vi "uPublisher BatchPublish.vi"(8 "error in (no error)":errorcluster, 10 "uMsgs":refnum<class "uMsg.lvclass">[](array[class]), 11 "uClient_Publisher in":refnum<class "uClient_Publisher.lvclass">) -> (0 "error out":errorcluster, 3 "uClient_Publisher out":refnum<class "uClient_Publisher.lvclass">)   [LabVIEW 2023, in "uLib.lvlib" / "uClient_Publisher.lvclass"]
doc: "Publish a batch of event to the broker in performance optimized manner."
uses:
  uClient_Publisher.lvclass
  uMsg/uMsg/uMsg.lvclass
  uClient_Publisher.lvclass/uClient_Publisher.ctl
  uData/uData/uData.lvclass
  uMsg/uMsg/uMsg.lvclass/uMsg.ctl
  uData/uData/uData.lvclass/uData.ctl
  uData/uData/Condition Tag Name.vi
  uData/uData/Blank Key Reserved String.vi
  uTransport/uTransport/uTransport.lvclass
  uStringManipulation/uStringManipulation/uStringManipulation.lvclass
  U:/Projects/uLib/Src/uFramework/uClient/uClient.lvclass
  U:/Projects/uLib/Src/uFramework/uClient_Publisher/uClient_Publisher.lvclass
  U:/Projects/uLib/Src/uFramework/uTransport/uTransport.lvclass
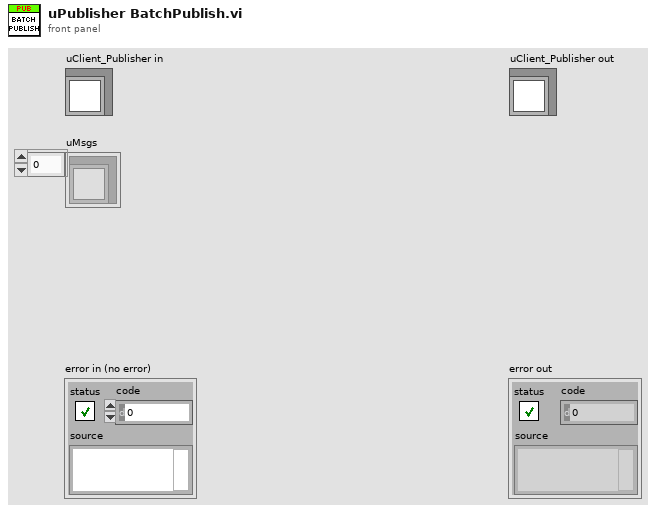
[diagram p1: front panel]
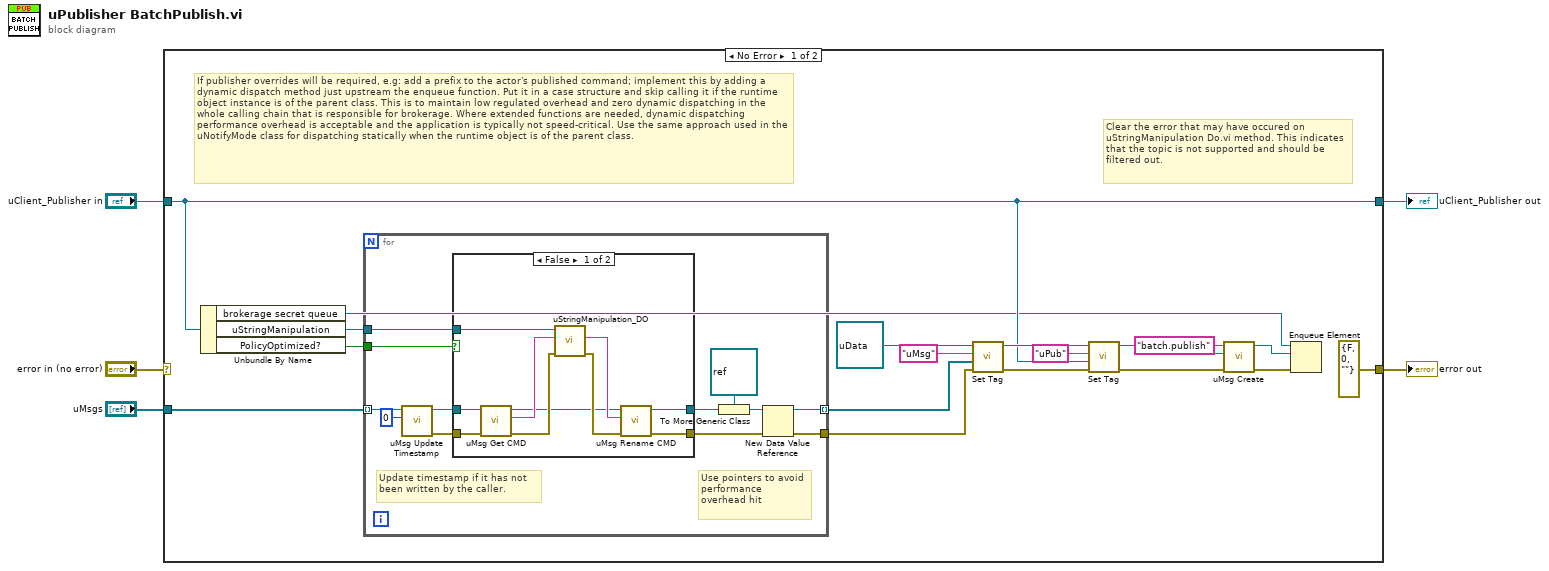
[diagram p0: block diagram]
diagram:
  n1 = case shown="No Error" "error in (no error)" {
    selector: "error in (no error)" -> [_ w48]
    tunnel: [errorcluster {"status"=FALSE, "code"=0, "source"=""} ("error IO") w48] -> w5
    tunnel: "uClient_Publisher in" -> [w12 w49]
    tunnel: "uMsgs" -> [w7 _]
    tunnel: [w12 w49] -> w2
    frame No Error {
      # "Clear the error that may have occured on uStringManipulation Do.vi method. This indicates that the topic is not supported and should be filtered out."
      # "If publisher overrides will be required, e.g: add a prefix to the actor's published command; implement this by adding a dynamic dispatch method just upstream the enqueue function. Put it in a case structure and skip calling it if the runtime object instance is of the parent class. This is to maintain low regulated overhead and zero dynamic dispatching in the whole calling chain that is responsible for brokerage. Where extended functions are needed, dynamic dispatching performance overhead is acceptable and the application is typically not speed-critical. Use the same approach used in the uNotifyMode class for dispatching statically when the runtime object is of the parent class."
      n2 = Unbundle By Name(w12) -> ("brokerage secret queue"=w6:refnum<queue>, "uStringManipulation"=w13:refnum<class "uStringManipulation.lvclass">, "PolicyOptimized?"=w8:bool)
      n3 = for {
        tunnel: [w35] -> w15
        tunnel: [w28] -> w14 mode=indexing
        tunnel: w13 -> [w34]
        tunnel: w8 -> [w33]
        tunnel: w7 -> [w30] mode=indexing
        # "Use pointers to avoid performance overhead hit"
        # "Update timestamp if it has not been written by the caller."
        n4 = call "uMsg Update Timestamp.vi"("Timestamp"=u32 0, "uMsg in"=w30) -> ("error out"=w29:errorcluster, "uMsg out"=w31:refnum<class "uMsg.lvclass">)  [unwired: 8 in]
        n5 = case shown="False" w33 {
          tunnel: w34 -> [w45 _]
          tunnel: w31 -> [w42 w47]
          tunnel: [w43 w47] -> w27
          tunnel: w29 -> [w38 w46]
          tunnel: [w36 w46] -> w24
          frame False {
            n6 = call "uMsg Get CMD.vi"("error in (no error)"=w38, "uMsg in"=w42) -> ("error out"=w41:errorcluster, "CMD"=w39:string, "uMsg out"=w37:refnum<class "uMsg.lvclass">)  [unwired: 7 in]
            n7 = call-dynamic "uStringManipulation_DO.vi"("error in (no error)"=w41, "String in"=w39, "uStringManipulation in"=w45) -> ("error out"=w40:errorcluster, "String"=w44:string)  [unwired: 6 in, 1 out]
            n8 = call "uMsg Rename CMD.vi"("error in (no error)"=w40, "New CMD"=w44, "uMsg in"=w37) -> ("error out"=w36:errorcluster, "uMsg out"=w43:refnum<class "uMsg.lvclass">)  [unwired: 7 in]
          }
          frame True {
            # "Avoid the unnecessary dynamic dispatch uStringManipulation method's overhead  if there is no translation provided."
          }
        }
        n9 = To More Generic Class(target class=refnum<class> refnum ("LabVIEW Object"), reference=w27) -> (generic class reference=w26:refnum<class>)
        n10 = New Data Value Reference(data value=w26, error in=w24) -> (data value reference=w28:refnum<data-value>, error out=w35:errorcluster)
      }
      n11 = call "Set Tag.vi"("error in (no error)"=w15, "Variant"=w14, "tag (case insensitive)"="uMsg", "uData in"=refnum<class "uData.lvclass"> refnum) -> ("error out"=w21:errorcluster, "uData out"=w19:refnum<class "uData.lvclass">)  [unwired: 5 in, 1 out]
      n12 = call "Set Tag.vi"("error in (no error)"=w21, "Variant"=w12, "tag (case insensitive)"="uPub", "uData in"=w19) -> ("error out"=w23:errorcluster, "uData out"=w16:refnum<class "uData.lvclass">)  [unwired: 5 in, 1 out]
      n13 = call "uMsg Create.vi"("error in (no error)"=w23, "Payload"=w16, "CMD"="batch.publish") -> ("error out"=w9:errorcluster, "uMsg out"=w10:refnum<class "uMsg.lvclass">)  [unwired: 7 in]
      n14 = Enqueue Element(queue=w6, element=w10, error in (no error)=w9) -> ()  [unwired: 1 in, 3 out]
    }
    frame Error {
    }
  }
  "error out" <- w5
  "uClient_Publisher out" <- w2
